vi "Read Dual Fan Actor.vi"(11 "Simulated Cooler":refnum<class "Simulated Evaporative Cooler.lvclass">) -> (2 "Dual Fan":refnum<class "Dual Fan.lvclass">)   [LabVIEW 2018, in "Simulated Evaporative Cooler.lvclass"]
uses:
  Simulated Evaporative Cooler.lvclass
  Dual Fan/Dual Fan/Dual Fan.lvclass
  Simulated Dual Fan/Simulated Dual Fan.lvclass
  C:/GitClones/LGP5-Resources/Frameworks/Actor Framework/Feedback Evaporative Cooler/Dual Fan/Dual Fan/Dual Fan.lvclass
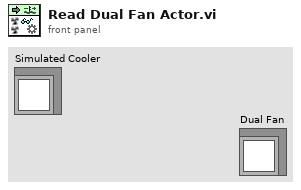
[diagram p1: front panel]
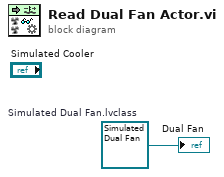
[diagram p0: block diagram]
diagram:
  w1 = refnum<class "Simulated Dual Fan.lvclass"> refnum  # Simulated Dual Fan.lvclass
  "Dual Fan" <- w1
